vi "Is Actor Class or Interface.vi"(6 "Validation":T1, 8 "error in (no error)":errorcluster, 10 "Target in":refnum<vi>, 11 "LVClass Library in":refnum<vi>) -> (0 "error out":errorcluster, 1 "is actor?":bool, 2 "TargetItem out":refnum<vi>, 4 "is actor interface?":bool)   [LabVIEW 2020, in "Message Maker.lvlib"]
uses:
  Message Maker.lvlib
  AFPP Shared/AFPP Shared.lvlib
  AFPP Shared/Validation Mode.ctl
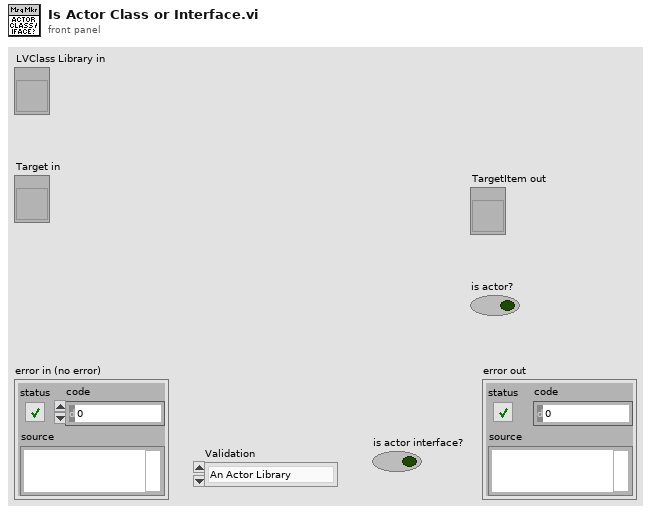
[diagram p1: front panel]
types:
  T1 = typedef "AFPP Shared.lvlib/Validation Mode.ctl" = enum16{"An Actor Library", "A Target Tag"}
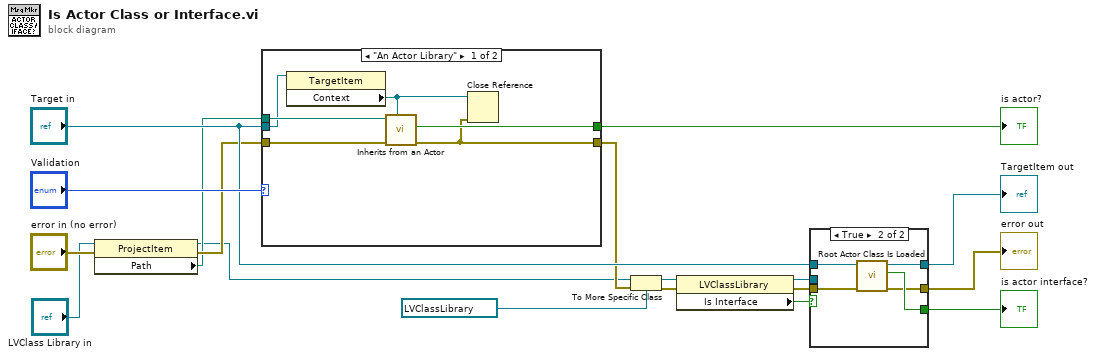
[diagram p0: block diagram]
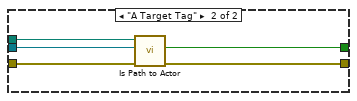
[diagram p2: hidden frame]
diagram:
  n1 = property class="ProjectItem"(reference="LVClass Library in", error in="error in (no error)") -> (reference out=w1:refnum<vi>, error out=w4:errorcluster, "Path"=w3:path)
  n2 = case shown="\"An Actor Library\"" "Validation" {
    tunnel: w4 -> [w23 w29]
    tunnel: [w20 w28] -> w6
    tunnel: w3 -> [w24 w27]
    tunnel: [w22 w26] -> w11
    tunnel: "Target in" -> [w21 w25]
    frame "An Actor Library" {
      n3 = property class="TargetItem"(reference=w21) -> ("Context"=w19:refnum<vi>)  [unwired: 1 in, 2 out]
      n4 = call "Inherits from an Actor.vi"("App Reference (this app)"=w19, "error in (no error)"=w23, "Path"=w24) -> ("error out"=w20:errorcluster, "Is Path to Actor?"=w22:bool)  [unwired: 6 in, 1 out]
      n5 = Close Reference(reference=w19, error in (no error)=w20) -> ()  [unwired: 1 out]
    }
    frame "A Target Tag" {
      n6 = call "Is Path to Actor.vi"("error in (no error)"=w29, "Target"=w25, "Path"=w27) -> ("error out"=w28:errorcluster, "Is Path to Actor?"=w26:bool)  [unwired: 6 in, 1 out]
    }
  }
  "is actor?" <- w11
  n7 = To More Specific Class(target class=refnum<vi> refnum ("LVClassLibrary in"), reference=w1, error in=w6) -> (specific class reference=w8:refnum<vi>, error out=w7:errorcluster)
  n8 = property class="LVClassLibrary"(reference=w8, error in=w7) -> (reference out=w13:refnum<vi>, error out=w17:errorcluster, "Is Interface"=w14:bool)
  n9 = case shown="True" w14 {
    tunnel: w13 -> [_ _]
    tunnel: [_ w34] -> w15
    tunnel: "Target in" -> [w31 w36]
    tunnel: [w31 w35] -> w16
    tunnel: w17 -> [w30 w33]
    tunnel: [w30 w32] -> w18
    frame False {
    }
    frame True {
      n10 = call "Root Actor Class Is Loaded.vi"("error in (no error)"=w33, "TargetItem in"=w36) -> ("error out"=w32:errorcluster, "is Actor.lvclass loaded already?"=w34:bool, "TargetItem out"=w35:refnum<vi>)  [unwired: 7 in]
    }
  }
  "error out" <- w18
  "TargetItem out" <- w16
  "is actor interface?" <- w15
